vi "ELSend.vi"(1 "DEOJ":string="013501", 2 "SEOJ":string="05FF01", 3 "EDT":string="30", 4 "EPC":string="80", 5 "ESV":string="60", 6 "IP address":string="224.0.23.0") -> (0 "Error Out":errorcluster caption="エラー出力")   [LabVIEW 2014]
uses:
  <vilib>/Utility/tcp.llb/UDP Multicast Write-Only Open.vi
panel:
  out "PDC":string
  out "OPC":string
  in  "TID":string="0000"
  in  "EDT 1":string(combo)="30"
  in  "EPC:構成プロパティ 4":string(combo)="80"
  in  "EDT 4":string(combo)="30"
  in  "EDT 3":string(combo)="30"
  in  "EPC:構成プロパティ 3":string(combo)="80"
  in  "EDT 2":string(combo)="30"
  in  "EPC:構成プロパティ 2":string(combo)="80"
  in  "EPC:構成プロパティ１":string(combo)="80"
  in  "DEOJ":string(combo)="0130"
  in  "SEOJ":string(combo)="05ff"
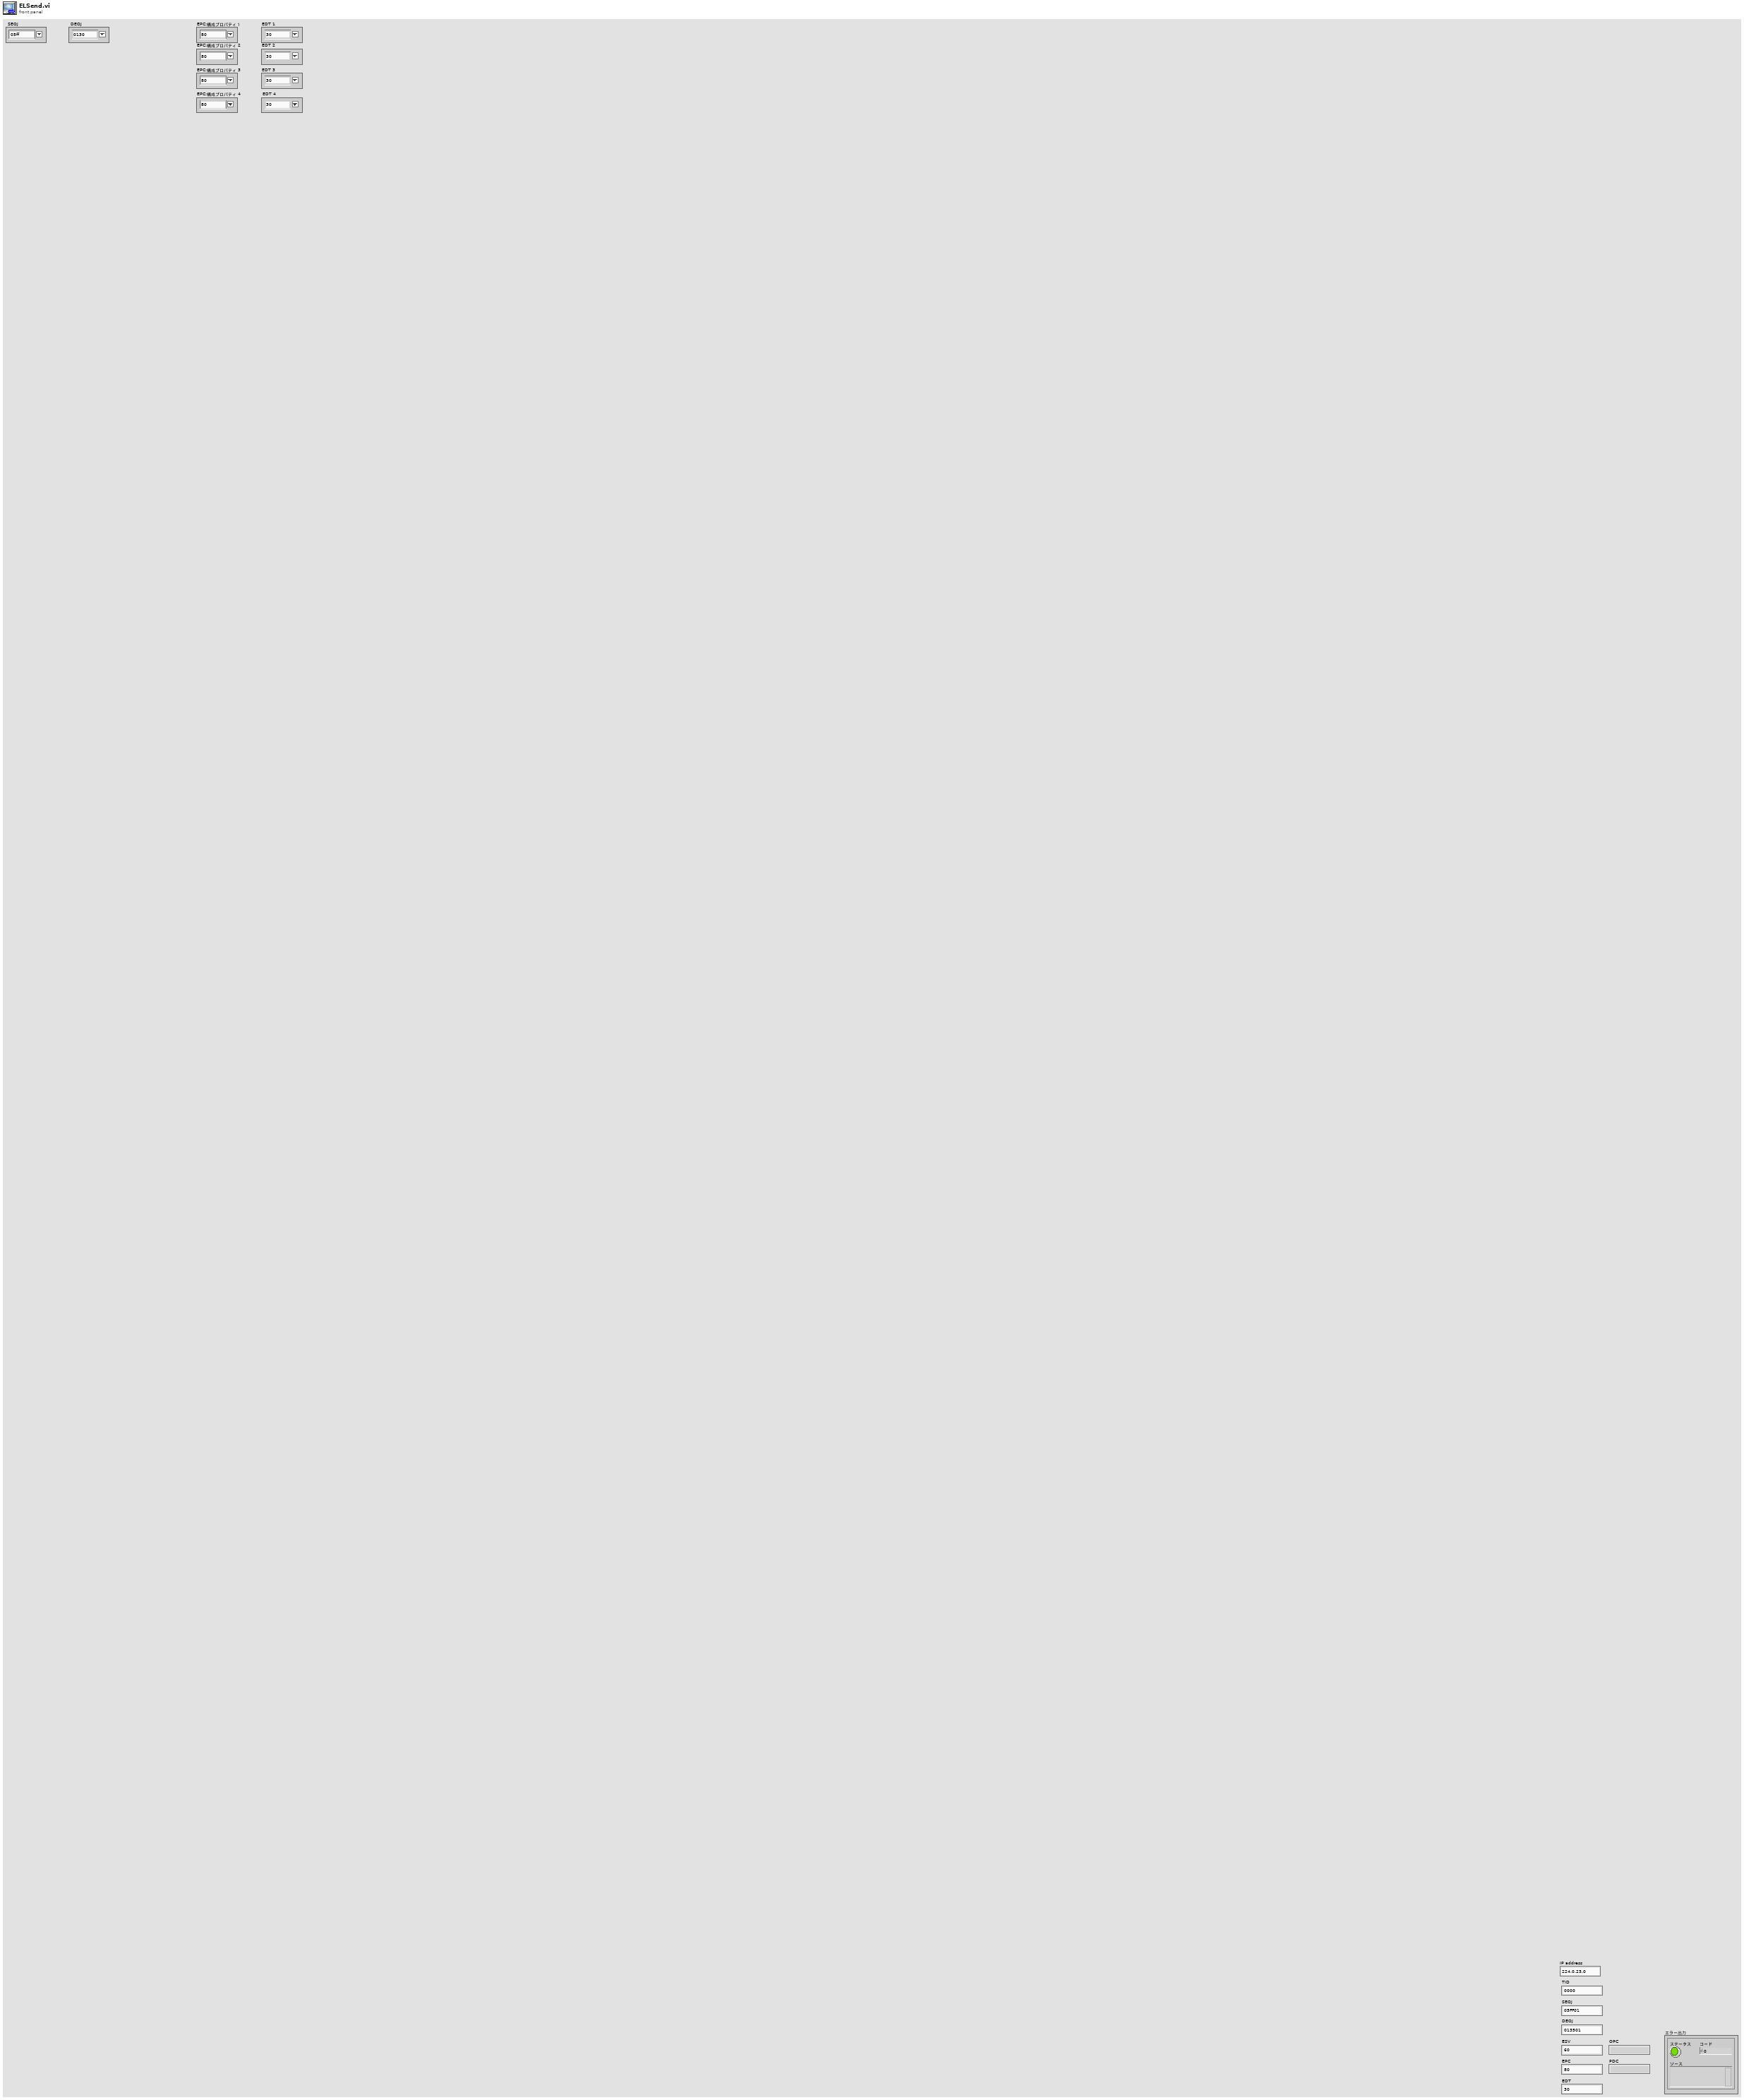
[diagram p1: front panel]
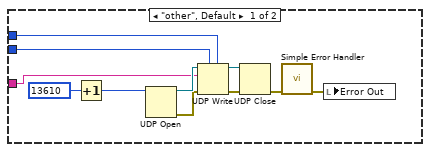
[diagram p3: hidden frame]
diagram:
  w2 = "01"
  n1 = String Length(string="EDT") -> (length=w10:i32)
  n2 = Divide(x=w10, y=2) -> (x/y=w9:dbl)
  n3 = Number To Hexadecimal String(1:2, 2:w9) -> (0:w1:string)
  "PDC" <- w1
  n4 = Concatenate Strings("1081", "TID", "SEOJ", "DEOJ", "ESV", w2, "EPC", w1, "EDT") -> (w4:string)
  n5 = flat-sequence {
    tunnel: w4 -> [w20]
    tunnel: [w19] -> w3
    frame #0 {
      # "String to HEX"
      n6 = String Length(string=w20) -> (length=w24:i32)
      n7 = Quotient & Remainder(x=w24, y=2) -> (x-y*floor(x/y)=w22:i32, floor(x/y)=w26:i32)
      n8 = Equal To 0?(x=w22) -> (x = 0?=w21:bool)
      n9 = case shown="False" w21 {
        tunnel: w26 -> [w29 w30]
        tunnel: [w28 w30] -> w23
        frame False {
          n10 = Increment(x=w29) -> (x+1=w28:i32)
        }
        frame True {
        }
      }
      n11 = for "Forループ" {
        N: w23 -> [_]
        tunnel: w20 -> [w40]
        shift-right: [w31] -> w19
        shift-left: "" -> [w33]
        i -> [w41]
        w38 = 2 ("x")
        n12 = Multiply(x=w38, y=w41) -> (x*y=w39:i32)
        n13 = String Subset(string=w40, offset (0)=w39, length (rest)=w38) -> (substring=w32:string)
        n14 = Hexadecimal String To Number(string=w32) -> (number=w37:u32)  [unwired: 2 in, 1 out]
        n15 = Build Array ("配列連結\n追加")(w37) -> (w34:u32[])
        n16 = To Unsigned Byte Integer(number=w34) -> (unsigned 8bit integer=w35:u8[])
        n17 = Byte Array To String ("バイト配列を\n文字列に変換")(unsigned byte array=w35) -> (string=w36:string)
        n18 = Concatenate Strings(w33, w36) -> (w31:string)
      }
    }
  }
  n19 = String To IP(1:"IP address") -> (0:w6:u32)
  n20 = case shown="\"224.0.23.0\"" "IP address" {
    tunnel: w3 -> [w42 w55]
    tunnel: w6 -> [w44 w53]
    tunnel: 3610 -> [w43 w54]
    frame "other", Default {
      n21 = Increment(x=13610) -> (x+1=w48:i32)
      n22 = UDP Open(11:w48) -> (port=w47:refnum<k16>, 0:w46:errorcluster)  [unwired: 4 in, 1 out]
      n23 = UDP Write(address=w44, port or service name=w43, connection ID=w47, data in=w42, 8:w46) -> (error out=w52:errorcluster, 3:w51:refnum<k16>)  [unwired: 1 in]
      n24 = UDP Close(connection ID=w51, 8:w52) -> (error out=w50:errorcluster)  [unwired: 1 out]
      n25 = call <vilib>:"Simple Error Handler.vi"("error in (no error)"=w50) -> ("error out"=w45:errorcluster)  [unwired: 4 in, 4 out]
      n26 = local write "Error Out"(w45) -> ()
    }
    frame "224.0.23.0" {
      n27 = Increment(x=13610) -> (x+1=w60:i32)
      n28 = call-poly <vilib>:"UDP Multicast Open.vi"("port"=w60) -> ("error out"=w61:errorcluster, "connection ID"=w62:refnum<k16>)  [unwired: 9 in]
      n29 = UDP Write(address=w53, port or service name=w54, connection ID=w62, data in=w55, 8:w61) -> (error out=w56:errorcluster, 3:w57:refnum<k16>)  [unwired: 1 in]
      n30 = UDP Close(connection ID=w57, 8:w56) -> (error out=w58:errorcluster)  [unwired: 1 out]
      n31 = call <vilib>:"Simple Error Handler.vi"("error in (no error)"=w58) -> ("error out"=→"Error Out":errorcluster)  [unwired: 4 in, 4 out]
    }
  }
  "OPC" <- w2
